vi "满度标定完成.vi"() -> ()   [LabVIEW 2013]
panel:
  in  "满度标定完成":bool
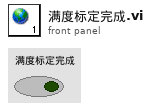
[diagram p1: front panel]
diagram:
